vi "Teleop.vi"(10 "Match Info":T1={"Autonomous Elapsed Seconds"=0.0, "TeleOp Elapsed Seconds"=0.0, "Disabled Elapsed Seconds"=0.0, "Visited Autonomous"=FALSE, "Visited TeleOp"=FALSE, "Visited Disabled"=FALSE, "Autonomous Settings"={"Autonomous Style"=enum."Independent", "VI Refnum"=refnum}}, 11 "Call Context":T2) -> ()   [LabVIEW 2012]
doc: "This VI is called for each TeleOp packet received from the DS where the robot is not disabled. It is often used to read from the joysticks and update I/O or to update setpoints for timed control loops. It should complete and return within 20 milliseconds or it may miss DS packets."
uses:
  <vilib>/Rock Robotics/WPI/DriverStation/WPI_DriverStationDerivedRobotMode.ctl
  <vilib>/Rock Robotics/WPI/DriverStation/WPI_DriverStationMatch Info.ctl
  <vilib>/Rock Robotics/WPI/Relay/WPI_RelayValue.ctl
  Robot Global Data.vi
  <vilib>/Rock Robotics/WPI/Joystick/WPI_JoystickGetSetRefNum.vi
panel:
  in  "Ext Const":dbl=0.5
  in  "Dep Const":dbl=1.0
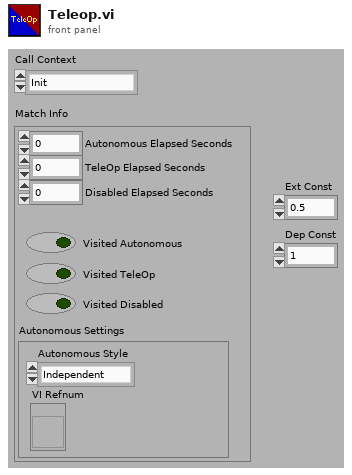
[diagram p1: front panel]
types:
  T1 = typedef "WPI_DriverStationMatch Info.ctl" = cluster{"Autonomous Elapsed Seconds":dbl, "TeleOp Elapsed Seconds":dbl, "Disabled Elapsed Seconds":dbl, "Visited Autonomous":bool, "Visited TeleOp":bool, "Visited Disabled":bool, "Autonomous Settings":cluster{"Autonomous Style":enum16{"Iterative", "Independent"}, "VI Refnum":refnum<vi>}}
  T2 = typedef "WPI_DriverStationDerivedRobotMode.ctl" = enum16{"Init", "Execute", "Stop"}
  T3 = typedef "WPI_RelayValue.ctl" = enum16{"Off", "On", "Forward", "Reverse"}
  T4 = cluster{"Driver Station Digital Input (1-8)[0]":bool, "Driver Station Digital Input (1-8)[1]":bool, "Driver Station Digital Input (1-8)[2]":bool, "Driver Station Digital Input (1-8)[3]":bool, "Driver Station Digital Input (1-8)[4]":bool, "Driver Station Digital Input (1-8)[5]":bool, "Driver Station Digital Input (1-8)[6]":bool, "Driver Station Digital Input (1-8)[7]":bool, "Driver Station Digital Input (1-8)[8]":bool}
  T5 = cluster{"Right Servo High":dbl, "Right Servo Mid":dbl, "Right Servo Low":dbl, "Left Servo High":dbl, "Left Servo Mid":dbl, "Left Servo Low":dbl}
  T6 = typedef "WPI_DigitalInputDevRef.ctl" = cluster{"DevStatus":errorcluster, "DIO Channel":T7, "Digital Module":T8}
  T7 = typedef "FPGA_DIOChannel.ctl" = enum8{"DIO 1", "DIO 2", "DIO 3", "DIO 4", "DIO 5", "DIO 6", "DIO 7", "DIO 8", "DIO 9", "DIO 10", "DIO 11", "DIO 12", "DIO 13", "DIO 14", "Invalid"}
  T8 = typedef "FPGA_TypedefDigitalModule.ctl" = enum16{"Digital Module 1", "Digital Module 2"}
  T9 = typedef "WPI_JoystickDevRef.ctl" = cluster{"Device":T10}
  T10 = typedef "WPI_JoystickDeviceEnum.ctl" = enum16{"USB 1", "USB 2", "USB 3", "USB 4", "Kinect 1", "Kinect 2"}
  T11 = cluster{"axis 1 (x)":dbl, "axis 2 (y)":dbl, "axis 3 (throttle)":dbl, "axis 4":dbl, "axis 5":dbl, "axis 6":dbl}
  T12 = typedef "WPI_ServoDeviceRef.ctl" = cluster{"DeviceStatus":errorcluster, "Digital Module":T8, "PWM Channel":T13, "DeadBand":T14}
  T13 = typedef "FPGA_DIOPWMChannel.ctl" = enum8{"PWM 1", "PWM 2", "PWM 3", "PWM 4", "PWM 5", "PWM 6", "PWM 7", "PWM 8", "PWM 9", "PWM 10", "Invalid"}
  T14 = typedef "WPI_PWMDeadband.ctl" = cluster{"Name":string, "maxPositivePwm":i32, "minPositivePwm":i32, "centerPwm":i32, "maxNegativePwm":i32, "minNegativePwm":i32, "angularRange":u16}
  T15 = typedef "WPI_RelayDevRef.ctl" = cluster{"DevStatus":errorcluster, "Relay Channel":T16, "Digital Module":T8, "Relay Direction":T17}
  T16 = typedef "FPGA_DIORelayChannel.ctl" = enum8{"Relay 1", "Relay 2", "Relay 3", "Relay 4", "Relay 5", "Relay 6", "Relay 7", "Relay 8", "Invalid"}
  T17 = typedef "WPI_RelayDirection.ctl" = enum16{"Both directions", "Forward only", "Reverse only"}
  T18 = typedef "WPI_MotorControlDeviceRef.ctl" = cluster{"DeviceStatus":errorcluster, "Type":enum16{"PWM", "CAN"}, "PWM":cluster{"Digital Module":T8, "PWM Channel":T13, "DeadBand":T14}, "CAN":cluster{"Device Number":u8, "Control Mode":T19, "Semaphore":T20, "Max Vout":dbl}, "Invert":bool, "TransformRef":T21, "InvTransformRef":T21}
  T19 = typedef "WPI_CANJaguar_ControlMode.ctl" = enum8{"Percent VBus", "Current", "Speed", "Position", "Voltage"}
  T20 = typedef "Semaphore RefNum" = refnum<k1>
  T21 = typedef "WPI_PWMTransform_ConPane.ctl" = refnum<vi>
  T22 = typedef "WPI_JoystickButtonState.ctl" = cluster{"Button 1":bool, "Button 2":bool, "Button 3":bool, "Button 4":bool, "Button 5":bool, "Button 6":bool, "Button 7":bool, "Button 8":bool, "Button 9":bool, "Button 10":bool, "Button 11":bool, "Button 12":bool}
  T23 = cluster{"FlipperLeftUp":dbl, "FlipperLeftDown":dbl, "FlipperRightUp":dbl, "FlipperRightDown":dbl, "KickerLeftBack":dbl, "KickerLeftForward":dbl, "KickerRightBack":dbl, "KickerRightForward":dbl}
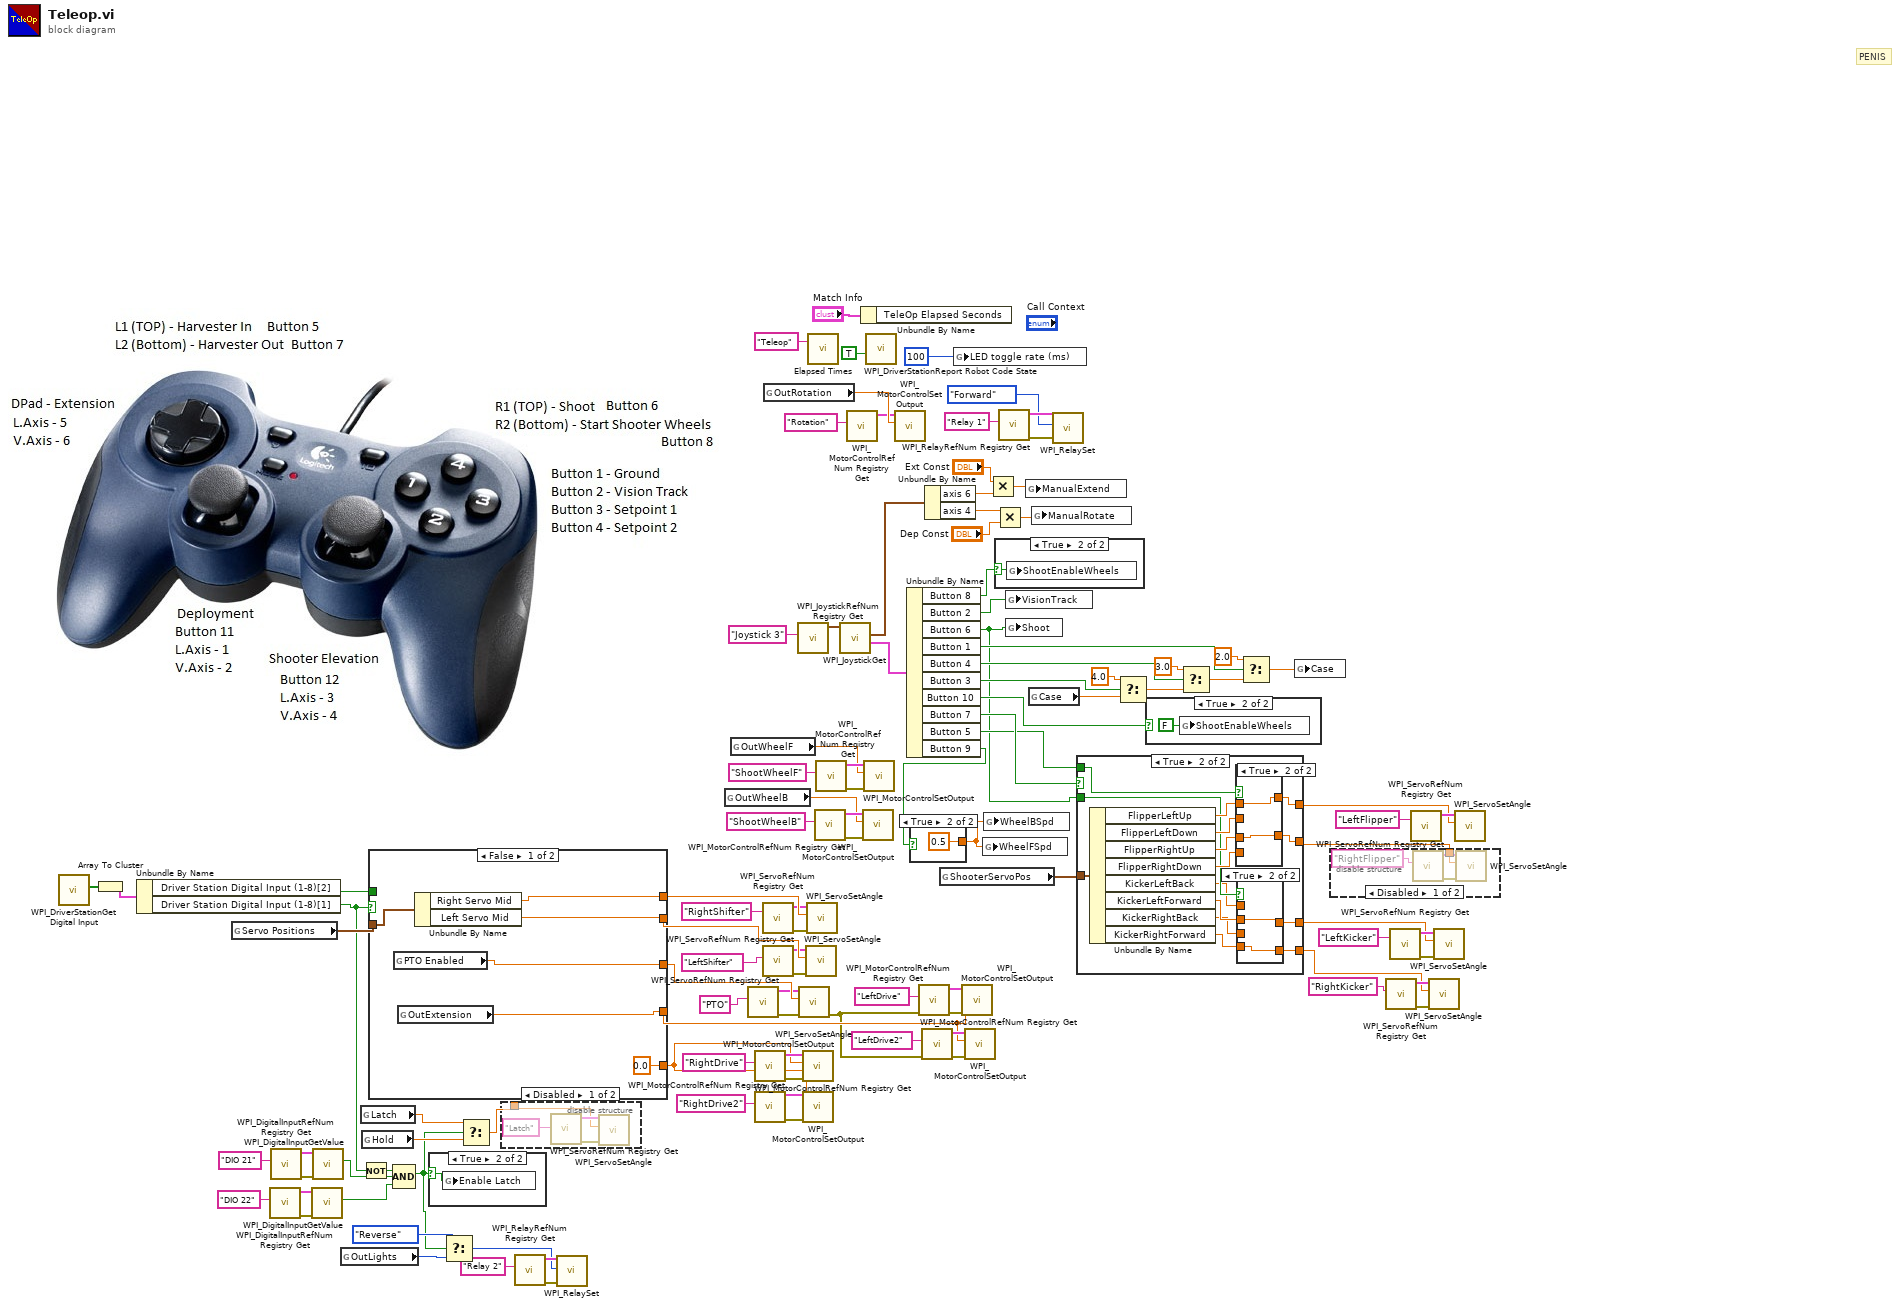
[diagram p0: block diagram]
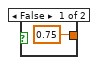
[diagram p3: hidden frame]
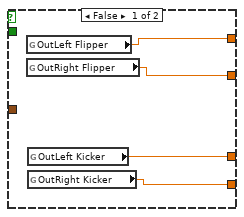
[diagram p5: hidden frame]
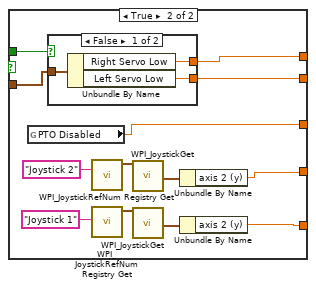
[diagram p9: hidden frame]
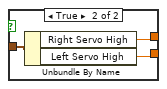
[diagram p10: hidden frame]
diagram:
  # "PENIS"
  n1 = call <vilib>:"WPI_DriverStationGet Digital Input.vi"() -> ("Driver Station Digital Input (1-8)"=w79:bool[])  [unwired: 11 in]
  n2 = Array To Cluster(array=w79) -> (cluster=w78:T4)
  n3 = Unbundle By Name(w78) -> ("Driver Station Digital Input (1-8)[2]"=w77:bool, "Driver Station Digital Input (1-8)[1]"=w41:bool)
  n4 = global read "Robot Global Data.vi" "Servo Positions"() -> (w76:T5)
  n5 = call <vilib>:"WPI_DigitalInputRefNum Registry Get.vi"("refnum name"="DIO 22") -> ("error out"=w5:errorcluster, "DigitalInputDevRef"=w6:T6)  [unwired: 9 in]
  n6 = call <vilib>:"WPI_DigitalInputRefNum Registry Get.vi"("refnum name"="DIO 21") -> ("error out"=w10:errorcluster, "DigitalInputDevRef"=w9:T6)  [unwired: 9 in]
  n7 = call <vilib>:"WPI_DigitalInputGetValue.vi"("error in (no error)"=w5, "DigitalInputDevRef"=w6) -> ("Value"=w2:bool)  [unwired: 7 in, 2 out]
  n8 = call <vilib>:"WPI_DigitalInputGetValue.vi"("error in (no error)"=w10, "DigitalInputDevRef"=w9) -> ("Value"=w3:bool)  [unwired: 7 in, 2 out]
  n9 = global read "Robot Global Data.vi" "OutLights"() -> (w44:T3)
  n10 = global read "Robot Global Data.vi" "Latch"() -> (w14:dbl)
  n11 = Not(x=w41) -> (.not. x?=w4:bool)
  n12 = global read "Robot Global Data.vi" "Hold"() -> (w13:dbl)
  n13 = case shown="False" w41 {
    tunnel: w77 -> [_ w130]
    tunnel: w76 -> [w117 w129]
    tunnel: [w116 w128] -> w75
    tunnel: [w115 w127] -> w74
    tunnel: [w114 w126] -> w67
    tunnel: [w112 w119] -> w66
    tunnel: [0.0 w118] -> w65
    frame False {
      n14 = global read "Robot Global Data.vi" "PTO Enabled"() -> (w114:dbl)
      n15 = global read "Robot Global Data.vi" "OutExtension"() -> (w112:dbl)
      n16 = Unbundle By Name(w117) -> ("Right Servo Mid"=w116:dbl, "Left Servo Mid"=w115:dbl)
    }
    frame True {
      n17 = global read "Robot Global Data.vi" "PTO Disabled"() -> (w126:dbl)
      n18 = case shown="False" w130 {
        tunnel: w129 -> [w133 w136]
        tunnel: [w132 w135] -> w128
        tunnel: [w131 w134] -> w127
        frame False {
          n19 = Unbundle By Name(w133) -> ("Right Servo Low"=w132:dbl, "Left Servo Low"=w131:dbl)
        }
        frame True {
          n20 = Unbundle By Name(w136) -> ("Right Servo High"=w135:dbl, "Left Servo High"=w134:dbl)
        }
      }
      n21 = call <vilib>:"WPI_JoystickRefNum Registry Get.vi"("refnum name"="Joystick 2") -> ("JoystickDevRef"=w120:T9)  [unwired: 1 in, 9 out]
      n22 = call <vilib>:"WPI_JoystickRefNum Registry Get.vi"("refnum name"="Joystick 1") -> ("JoystickDevRef"=w124:T9)  [unwired: 1 in, 9 out]
      n23 = call <vilib>:"WPI_JoystickGet.vi"("JoystickDevRef"=w120) -> ("Axes"=w122:T11)  [unwired: 1 in, 5 out]
      n24 = call <vilib>:"WPI_JoystickGet.vi"("JoystickDevRef"=w124) -> ("Axes"=w125:T11)  [unwired: 1 in, 5 out]
      n25 = Unbundle By Name(w122) -> ("axis 2 (y)"=w119:dbl)
      n26 = Unbundle By Name(w125) -> ("axis 2 (y)"=w118:dbl)
    }
  }
  n27 = Compound Arithmetic op=AND(w4, w3, w2) -> (w1:bool)
  n28 = case shown="True" w1 {
    selector: w1 -> [_ w137]
    frame False {
    }
    frame True {
      n29 = global write "Robot Global Data.vi" "Enable Latch"(w137) -> ()
    }
  }
  n30 = Select(t=WPI_RelayValue."Reverse" ("RelayValue"), s=w1, f=w44) -> (s? t:f=w42:T3)
  n31 = Select(t=w14, s=w1, f=w13) -> (s? t:f=w40:dbl)
  n32 = disable-structure shown="Disabled" {
    disable-tunnel: w40 -> [w138 _]
    frame Disabled {
      n33 = call <vilib>:"WPI_ServoRefNum Registry Get.vi"("refnum name"="Latch") -> ("error out"=w141:errorcluster, "ServoDeviceRef"=w139:T12)  [unwired: 9 in]
      n34 = call <vilib>:"WPI_ServoSetAngle.vi"("error in (no error)"=w141, "Angle"=w138, "ServoDeviceRef"=w139) -> ()  [unwired: 7 in, 2 out]
    }
    frame Enabled {
    }
  }
  n35 = call <vilib>:"WPI_RelayRefNum Registry Get.vi"("refnum name"="Relay 2") -> ("error out"=w50:errorcluster, "RelayDevRef"=w48:T15)  [unwired: 9 in]
  n36 = call <vilib>:"WPI_RelaySet.vi"("error in (no error)"=w50, "RelayValue"=w42, "RelayDevRef"=w48) -> ()  [unwired: 7 in, 2 out]
  n37 = global read "Robot Global Data.vi" "OutWheelB"() -> (w32:dbl)
  n38 = global read "Robot Global Data.vi" "OutWheelF"() -> (w33:dbl)
  n39 = call <vilib>:"WPI_ServoRefNum Registry Get.vi"("refnum name"="PTO") -> ("error out"=w60:errorcluster, "ServoDeviceRef"=w61:T12)  [unwired: 9 in]
  n40 = call <vilib>:"WPI_MotorControlRefNum Registry Get.vi"("refnum name"="RightDrive") -> ("error out"=w89:errorcluster, "MotorControlDevRef"=w91:T18)  [unwired: 9 in]
  n41 = call <vilib>:"WPI_MotorControlRefNum Registry Get.vi"("refnum name"="RightDrive2") -> ("error out"=w82:errorcluster, "MotorControlDevRef"=w80:T18)  [unwired: 9 in]
  n42 = call <vilib>:"WPI_ServoRefNum Registry Get.vi"("refnum name"="RightShifter") -> ("error out"=w70:errorcluster, "ServoDeviceRef"=w71:T12)  [unwired: 9 in]
  n43 = call <vilib>:"WPI_ServoRefNum Registry Get.vi"("refnum name"="LeftShifter") -> ("error out"=w72:errorcluster, "ServoDeviceRef"=w73:T12)  [unwired: 9 in]
  n44 = global read "Robot Global Data.vi" "OutRotation"() -> (w64:dbl)
  n45 = call <vilib>:"WPI_JoystickRefNum Registry Get.vi"("refnum name"="Joystick 3") -> ("JoystickDevRef"=w108:T9)  [unwired: 9 in, 1 out]
  n46 = call <vilib>:"WPI_ServoSetAngle.vi"("error in (no error)"=w60, "Angle"=w67, "ServoDeviceRef"=w61) -> ("error out"=w56:errorcluster)  [unwired: 7 in, 1 out]
  n47 = call <vilib>:"WPI_MotorControlSetOutput.vi"("error in (no error)"=w89, "Output"=w65, "MotorControlDevRef"=w91) -> ()  [unwired: 6 in, 3 out]
  n48 = call <vilib>:"WPI_MotorControlSetOutput.vi"("error in (no error)"=w82, "Output"=w65, "MotorControlDevRef"=w80) -> ()  [unwired: 6 in, 3 out]
  n49 = call <vilib>:"WPI_ServoSetAngle.vi"("error in (no error)"=w72, "Angle"=w74, "ServoDeviceRef"=w73) -> ()  [unwired: 7 in, 2 out]
  n50 = call <vilib>:"WPI_ServoSetAngle.vi"("error in (no error)"=w70, "Angle"=w75, "ServoDeviceRef"=w71) -> ()  [unwired: 7 in, 2 out]
  n51 = call "Elapsed Times.vi"("Call Name"="Teleop") -> ()  [unwired: 2 in, 1 out]
  n52 = call <vilib>:"WPI_MotorControlRefNum Registry Get.vi"("refnum name"="ShootWheelB") -> ("error out"=w35:errorcluster, "MotorControlDevRef"=w36:T18)  [unwired: 9 in]
  n53 = call <vilib>:"WPI_MotorControlRefNum Registry Get.vi"("refnum name"="ShootWheelF") -> ("error out"=w37:errorcluster, "MotorControlDevRef"=w34:T18)  [unwired: 9 in]
  n54 = call <vilib>:"WPI_JoystickGet.vi"("JoystickDevRef"=w108) -> ("Buttons"=w106:T22, "Axes"=w105:T11)  [unwired: 4 in, 1 out]
  n55 = call <vilib>:"WPI_MotorControlRefNum Registry Get.vi"("refnum name"="Rotation") -> ("MotorControlDevRef"=w62:T18)  [unwired: 9 in, 1 out]
  n56 = Unbundle By Name("Match Info") -> ()  [unwired: 1 out]
  n57 = call <vilib>:"WPI_MotorControlSetOutput.vi"("error in (no error)"=w35, "Output"=w32, "MotorControlDevRef"=w36) -> ()  [unwired: 6 in, 3 out]
  n58 = call <vilib>:"WPI_MotorControlSetOutput.vi"("error in (no error)"=w37, "Output"=w33, "MotorControlDevRef"=w34) -> ()  [unwired: 6 in, 3 out]
  n59 = call <vilib>:"WPI_DriverStationReport Robot Code State.vi"("TeleOp"=TRUE ("Autonomous")) -> ()  [unwired: 10 in, 1 out]
  n60 = call <vilib>:"WPI_MotorControlSetOutput.vi"("Output"=w64, "MotorControlDevRef"=w62) -> ()  [unwired: 7 in, 3 out]
  n61 = Unbundle By Name(w106) -> ("Button 8"=w93:bool, "Button 2"=w104:bool, "Button 6"=w16:bool, "Button 1"=w103:bool, "Button 4"=w101:bool, "Button 3"=w100:bool, "Button 10"=w31:bool, "Button 7"=w30:bool, "Button 5"=w29:bool, "Button 9"=w11:bool)
  n62 = case shown="True" w11 {
    tunnel: [0.75 0.5] -> w12
    frame False {
    }
    frame True {
    }
  }
  n63 = call <vilib>:"WPI_MotorControlRefNum Registry Get.vi"("error in (no error)"=w56, "refnum name"="LeftDrive") -> ("error out"=w84:errorcluster, "MotorControlDevRef"=w87:T18)  [unwired: 8 in]
  n64 = call <vilib>:"WPI_MotorControlRefNum Registry Get.vi"("error in (no error)"=w56, "refnum name"="LeftDrive2") -> ("error out"=w83:errorcluster, "MotorControlDevRef"=w85:T18)  [unwired: 8 in]
  n65 = Unbundle By Name(w105) -> ("axis 6"=w47:dbl, "axis 4"=w57:dbl)
  n66 = global read "Robot Global Data.vi" "ShooterServoPos"() -> (w17:T23)
  n67 = global write "Robot Global Data.vi" "LED toggle rate (ms)"(u32 100 ("LED ms toggle rate")) -> ()
  n68 = call <vilib>:"WPI_MotorControlSetOutput.vi"("error in (no error)"=w84, "Output"=w66, "MotorControlDevRef"=w87) -> ()  [unwired: 6 in, 3 out]
  n69 = call <vilib>:"WPI_MotorControlSetOutput.vi"("error in (no error)"=w83, "Output"=w66, "MotorControlDevRef"=w85) -> ()  [unwired: 6 in, 3 out]
  n70 = global write "Robot Global Data.vi" "WheelFSpd"(w12) -> ()
  n71 = global write "Robot Global Data.vi" "WheelBSpd"(w12) -> ()
  n72 = Multiply(x="Ext Const", y=w47) -> (x*y=w45:dbl)
  n73 = Multiply(x=w57, y="Dep Const") -> (x*y=w55:dbl)
  n74 = case shown="True" w93 {
    selector: w93 -> [_ w144]
    frame False {
    }
    frame True {
      n75 = global write "Robot Global Data.vi" "ShootEnableWheels"(w144) -> ()
    }
  }
  n76 = call <vilib>:"WPI_RelayRefNum Registry Get.vi"("refnum name"="Relay 1") -> ("error out"=w52:errorcluster, "RelayDevRef"=w54:T15)  [unwired: 9 in]
  n77 = global write "Robot Global Data.vi" "VisionTrack"(w104) -> ()
  n78 = global write "Robot Global Data.vi" "Shoot"(w16) -> ()
  n79 = global write "Robot Global Data.vi" "ManualExtend"(w45) -> ()
  n80 = global read "Robot Global Data.vi" "Case"() -> (w95:dbl)
  n81 = global write "Robot Global Data.vi" "ManualRotate"(w55) -> ()
  n82 = call <vilib>:"WPI_RelaySet.vi"("error in (no error)"=w52, "RelayValue"=WPI_RelayValue."Forward", "RelayDevRef"=w54) -> ()  [unwired: 7 in, 2 out]
  n83 = case shown="True" w30 {
    tunnel: w29 -> [_ w149]
    tunnel: [w148 w162] -> w20
    tunnel: [w147 w160] -> w19
    tunnel: [w146 w151] -> w18
    tunnel: [w145 w150] -> w15
    tunnel: w17 -> [_ w163]
    tunnel: w16 -> [_ w156]
    frame False {
      n84 = global read "Robot Global Data.vi" "OutLeft Flipper"() -> (w148:dbl)
      n85 = global read "Robot Global Data.vi" "OutRight Flipper"() -> (w147:dbl)
      n86 = global read "Robot Global Data.vi" "OutLeft Kicker"() -> (w146:dbl)
      n87 = global read "Robot Global Data.vi" "OutRight Kicker"() -> (w145:dbl)
    }
    frame True {
      n88 = Unbundle By Name(w163) -> ("FlipperLeftUp"=w161:dbl, "FlipperLeftDown"=w158:dbl, "FlipperRightUp"=w159:dbl, "FlipperRightDown"=w157:dbl, "KickerLeftBack"=w155:dbl, "KickerLeftForward"=w154:dbl, "KickerRightBack"=w153:dbl, "KickerRightForward"=w152:dbl)
      n89 = case shown="True" w149 {
        tunnel: [w169 w171] -> w162
        tunnel: w161 -> [_ w171]
        tunnel: [w168 w170] -> w160
        tunnel: w159 -> [_ w170]
        tunnel: w158 -> [w169 _]
        tunnel: w157 -> [w168 _]
        frame False {
        }
        frame True {
        }
      }
      n90 = case shown="True" w156 {
        tunnel: w155 -> [w165 _]
        tunnel: w154 -> [_ w166]
        tunnel: w153 -> [w164 _]
        tunnel: w152 -> [_ w167]
        tunnel: [w165 w166] -> w151
        tunnel: [w164 w167] -> w150
        frame False {
        }
        frame True {
        }
      }
    }
  }
  n91 = Select(t=4.0, s=w100, f=w95) -> (s? t:f=w99:dbl)
  n92 = case shown="True" w31 {
    frame False {
    }
    frame True {
      n93 = global write "Robot Global Data.vi" "ShootEnableWheels"(FALSE ("ShootStartWheels")) -> ()
    }
  }
  n94 = Select(t=3.0, s=w101, f=w99) -> (s? t:f=w97:dbl)
  n95 = Select(t=2.0, s=w103, f=w97) -> (s? t:f=w94:dbl)
  n96 = global write "Robot Global Data.vi" "Case"(w94) -> ()
  n97 = disable-structure shown="Disabled" {
    disable-tunnel: w19 -> [w173 _]
    frame Disabled {
      n98 = call <vilib>:"WPI_ServoRefNum Registry Get.vi"("refnum name"="RightFlipper") -> ("error out"=w176:errorcluster, "ServoDeviceRef"=w174:T12)  [unwired: 9 in]
      n99 = call <vilib>:"WPI_ServoSetAngle.vi"("error in (no error)"=w176, "Angle"=w173, "ServoDeviceRef"=w174) -> ()  [unwired: 7 in, 2 out]
    }
    frame Enabled {
    }
  }
  n100 = call <vilib>:"WPI_ServoRefNum Registry Get.vi"("refnum name"="RightKicker") -> ("error out"=w27:errorcluster, "ServoDeviceRef"=w25:T12)  [unwired: 9 in]
  n101 = call <vilib>:"WPI_ServoRefNum Registry Get.vi"("refnum name"="LeftKicker") -> ("error out"=w21:errorcluster, "ServoDeviceRef"=w22:T12)  [unwired: 9 in]
  n102 = call <vilib>:"WPI_ServoRefNum Registry Get.vi"("refnum name"="LeftFlipper") -> ("ServoDeviceRef"=w23:T12)  [unwired: 9 in, 1 out]
  n103 = call <vilib>:"WPI_ServoSetAngle.vi"("error in (no error)"=w27, "Angle"=w15, "ServoDeviceRef"=w25) -> ()  [unwired: 7 in, 2 out]
  n104 = call <vilib>:"WPI_ServoSetAngle.vi"("error in (no error)"=w21, "Angle"=w18, "ServoDeviceRef"=w22) -> ()  [unwired: 7 in, 2 out]
  n105 = call <vilib>:"WPI_ServoSetAngle.vi"("Angle"=w20, "ServoDeviceRef"=w23) -> ()  [unwired: 8 in, 2 out]
